vi "Voltage or Resistance.vi"(0 "Data In":fxp<+/-,28,17>[](array[numeric])=[0.0, 0.0, 0.0, 0.0, 0.0, 0.0, 0.0, 0.0, 0.0, 0.0, 0.0, 0.0, 0.0], 7 "Resistance In":fxp<+/-,28,17>[](array[numeric])=[0.0, 0.0, 0.0, 0.0, 0.0, 0.0, 0.0, 0.0, 0.0, 0.0], 11 "V(T)/R(F)":bool) -> (4 "Data Out":fxp<+/-,28,17>[](array[numeric]))   [LabVIEW 2013]
uses:
  <vilib>/rvi/FXPMathLib/FxpDiv/subVIs/nifxpmath_Div_SimConfig.ctl
  <vilib>/rvi/FXPMathLib/FxpDiv/simVIs/DllFxpDivTemp_sub.vi
  <vilib>/rvi/FXPMathLib/FxpSub/XNode/nifxpmath_Sub.xnode
  <vilib>/rvi/FXPMathLib/FxpDiv/XNode/nifxpmath_Div.xnode
  <vilib>/rvi/FXPMathLib/sim/FxpSim.dll
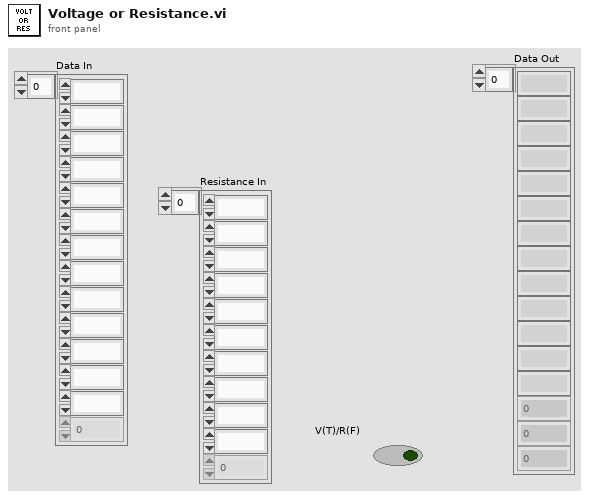
[diagram p1: front panel]
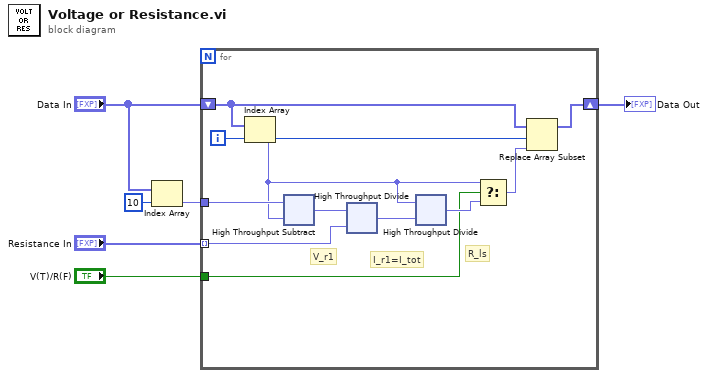
[diagram p0: block diagram]
diagram:
  n1 = Index Array(array="Data In", index=10) -> (element=w3:fxp<+/-,28,17>)
  n2 = for {
    tunnel: "Resistance In" -> [w12] mode=indexing
    shift-right: [w16] -> w2
    shift-left: "Data In" -> [w17]
    tunnel: w3 -> [w14]
    tunnel: "V(T)/R(F)" -> [w7]
    i -> [w15]
    # "R_ls"
    # "I_r1=I_tot"
    # "V_r1"
    n3 = Index Array(array=w17, index=w15) -> (element=w10:fxp<+/-,28,17>)
    n4 = xnode "High Throughput Subtract"("x"=w14, "y"=w10) -> ("x-y"=w13:fxp<+/-,29,18>)
    n5 = xnode "High Throughput Divide"("x"=w13, "y"=w12) -> ("x/y"=w11:fxp<+/-,29,8>)
    n6 = xnode "High Throughput Divide"("x"=w10, "y"=w11) -> ("x/y"=w9:fxp<+/-,28,17>)
    n7 = Select(t=w10, s=w7, f=w9) -> (s? t:f=w8:fxp<+/-,28,17>)
    n8 = Replace Array Subset(array=w17, new element=w8, index=w15) -> (w16:fxp<+/-,28,17>[])
  }
  "Data Out" <- w2
